vi "WriteZ.vi"(5 "new-z (um)":dbl, 7 "Method":u16(ring)=1 items=["Analogue", "Serial"], 8 "error in (no error)":errorcluster, 11 "ASI VISA resource name":refnum<visa-resource-name>) -> (0 "error out":errorcluster, 1 "V":dbl, 3 "ASI VISA resource name OUT":refnum<visa-resource-name>)   [LabVIEW 2018]
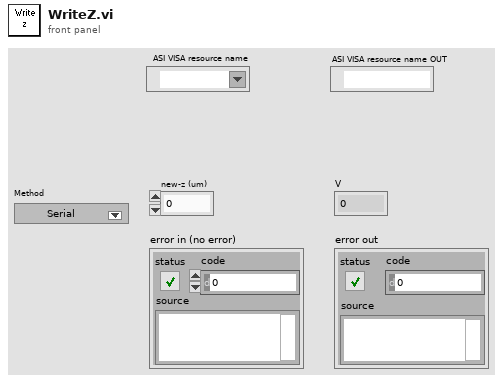
[diagram p1: front panel]
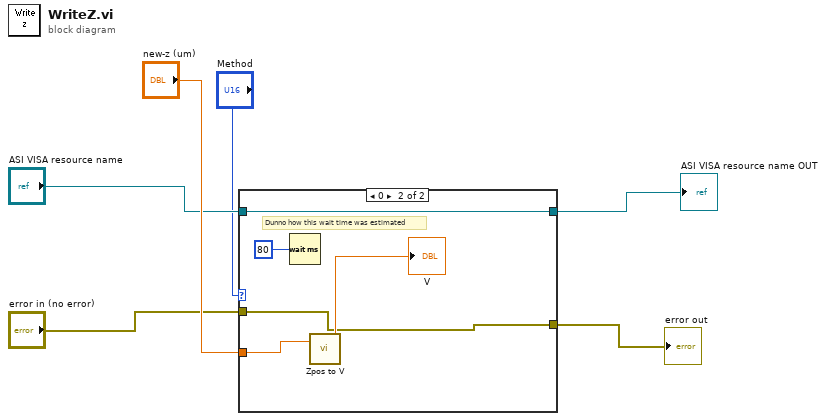
[diagram p0: block diagram]
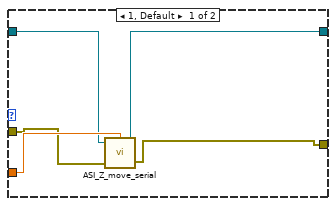
[diagram p2: hidden frame]
diagram:
  n1 = case shown="0" "Method" {
    tunnel: "new-z (um)" -> [w11 w16]
    tunnel: [w7 w12] -> w5
    tunnel: "error in (no error)" -> [w9 w12]
    tunnel: "ASI VISA resource name" -> [w10 w14]
    tunnel: [w8 w14] -> w1
    frame 1, Default {
      n2 = call "ASI_Z_move_serial.vi"("Z position (um)"=w11, "error in"=w9, "VISA resource name"=w10) -> ("error out"=w7:errorcluster, "VISA resource name out"=w8:refnum<visa-resource-name>)  [unwired: 1 in]
    }
    frame 0 {
      # "Dunno how this wait time was estimated"
      n3 = Wait (ms)(milliseconds to wait=u32 80) -> ()  [unwired: 1 out]
      n4 = call "Zpos to V.vi"("Z (um)"=w16) -> ("V"=→"V":dbl)  [unwired: 2 in]
    }
  }
  "error out" <- w5
  "ASI VISA resource name OUT" <- w1
